vi "Keyboard.vi"() -> ()   [LabVIEW 2018]
panel:
  out "Keys Output":u8[](array[numeric])
  in  "Keys":u8[](array[numeric])
  out "Char":i16 format="%x"
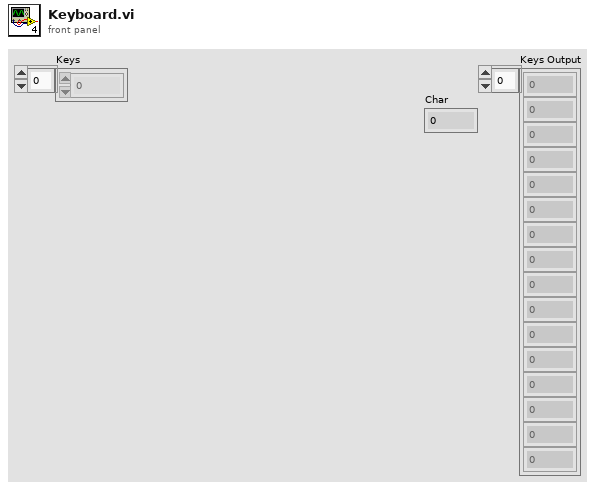
[diagram p1: front panel]
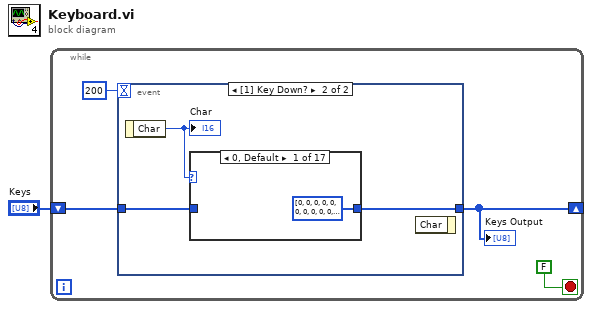
[diagram p0: block diagram]
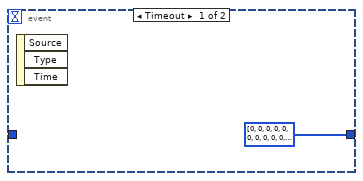
[diagram p2: hidden frame]
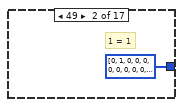
[diagram p3: hidden frame]
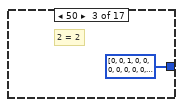
[diagram p4: hidden frame]
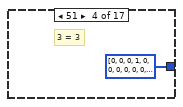
[diagram p5: hidden frame]
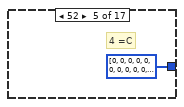
[diagram p6: hidden frame]
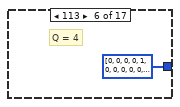
[diagram p7: hidden frame]
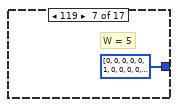
[diagram p8: hidden frame]
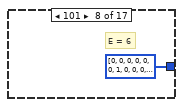
[diagram p9: hidden frame]
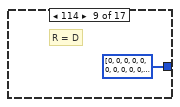
[diagram p10: hidden frame]
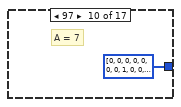
[diagram p11: hidden frame]
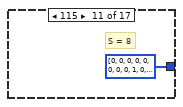
[diagram p12: hidden frame]
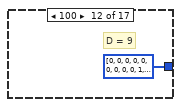
[diagram p13: hidden frame]
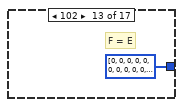
[diagram p14: hidden frame]
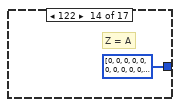
[diagram p15: hidden frame]
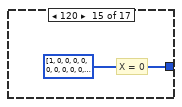
[diagram p16: hidden frame]
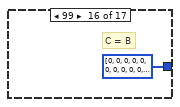
[diagram p17: hidden frame]
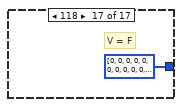
[diagram p18: hidden frame]
diagram:
  n1 = while {
    shift-right: [w3] -> _
    shift-left: "Keys" -> [w4]
    stop <- FALSE stop-if-true
    n2 = event shown="[1] Key Down?" {
      selector: _ -> [_ _]
      dyn-events: _ -> [_ _]
      timeout: 200 -> [_ _]
      tunnel: w4 -> [_ w8]
      tunnel: [u8[] [0, 0, 0, 0, 0, 0, 0, 0, 0, 0, 0, 0, 0, 0, 0, 0, 0] ("Keys 2") w7] -> w3
      event Timeout {
        n3 = event-data() -> ()  [unwired: 1 in, 3 out]
      }
      event Key Down? {
        n4 = event-data() -> ("Char"=w9:i16)  [unwired: 1 in]
        "Char" <- w9
        n5 = case shown="0, Default" w9 {
          tunnel: [u8[] [0, 0, 0, 0, 0, 0, 0, 0, 0, 0, 0, 0, 0, 0, 0, 0] ("Keys 2") u8[] [0, 1, 0, 0, 0, 0, 0, 0, 0, 0, 0, 0, 0, 0, 0, 0] ("Keys 2") u8[] [0, 0, 1, 0, 0, 0, 0, 0, 0, 0, 0, 0, 0, 0, 0, 0] ("Keys 2") u8[] [0, 0, 0, 1, 0, 0, 0, 0, 0, 0, 0, 0, 0, 0, 0, 0] ("Keys 2") u8[] [0, 0, 0, 0, 0, 0, 0, 0, 0, 0, 0, 0, 1, 0, 0, 0] ("Keys 2") u8[] [0, 0, 0, 0, 1, 0, 0, 0, 0, 0, 0, 0, 0, 0, 0, 0] ("Keys 2") u8[] [0, 0, 0, 0, 0, 1, 0, 0, 0, 0, 0, 0, 0, 0, 0, 0] ("Keys 2") u8[] [0, 0, 0, 0, 0, 0, 1, 0, 0, 0, 0, 0, 0, 0, 0, 0] ("Keys 2") u8[] [0, 0, 0, 0, 0, 0, 0, 0, 0, 0, 0, 0, 0, 1, 0, 0] ("Keys 2") u8[] [0, 0, 0, 0, 0, 0, 0, 1, 0, 0, 0, 0, 0, 0, 0, 0] ("Keys 2") u8[] [0, 0, 0, 0, 0, 0, 0, 0, 1, 0, 0, 0, 0, 0, 0, 0] ("Keys 2") u8[] [0, 0, 0, 0, 0, 0, 0, 0, 0, 1, 0, 0, 0, 0, 0, 0] ("Keys 2") u8[] [0, 0, 0, 0, 0, 0, 0, 0, 0, 0, 0, 0, 0, 0, 1, 0] ("Keys 2") u8[] [0, 0, 0, 0, 0, 0, 0, 0, 0, 0, 1, 0, 0, 0, 0, 0] ("Keys 2") u8[] [1, 0, 0, 0, 0, 0, 0, 0, 0, 0, 0, 0, 0, 0, 0, 0] ("Keys 2") u8[] [0, 0, 0, 0, 0, 0, 0, 0, 0, 0, 0, 1, 0, 0, 0, 0] ("Keys 2") u8[] [0, 0, 0, 0, 0, 0, 0, 0, 0, 0, 0, 0, 0, 0, 0, 1] ("Keys 2")] -> w7
          tunnel: w8 -> [_ _ _ _ _ _ _ _ _ _ _ _ _ _ _ _ _]
          frame 0, Default {
          }
          frame 49 {
            # "1 = 1"
          }
          frame 50 {
            # "2 = 2"
          }
          frame 51 {
            # "3 = 3"
          }
          frame 52 {
            # "4 =C"
          }
          frame 113 {
            # "Q = 4"
          }
          frame 119 {
            # "W = 5"
          }
          frame 101 {
            # "E = 6"
          }
          frame 114 {
            # "R = D"
          }
          frame 97 {
            # "A = 7"
          }
          frame 115 {
            # "S = 8"
          }
          frame 100 {
            # "D = 9"
          }
          frame 102 {
            # "F = E"
          }
          frame 122 {
            # "Z = A"
          }
          frame 120 {
            # "X = 0"
          }
          frame 99 {
            # "C = B"
          }
          frame 118 {
            # "V = F"
          }
        }
        n6 = event-data() -> ()  [unwired: 2 in, 1 out]
      }
    }
    "Keys Output" <- w3
  }
